vi "UTILITY Get Excel Data From Worksheet.vi"(8 "error in (no error)":errorcluster, 10 "Number of Columns":i32, 11 "template (empty)":path) -> (0 "error out":errorcluster, 3 "Array":string[][](array[string]))   [LabVIEW 2016]
uses:
  <vilib>/addons/_office/excel.llb/Excel Get Data (str).vi
  <vilib>/Utility/NIReport.llb/NI_report.lvclass
  <vilib>/Utility/NIReport.llb/Excel/NI_Excel.lvclass
  <vilib>/addons/_office/NI_ReportGenerationToolkit.lvlib
panel:
  in  "start (0, 0) 2":cluster{"start row":i32, "start column":i32}
  out "MS Office parameters out 2":T1
  # "Input the file to read"
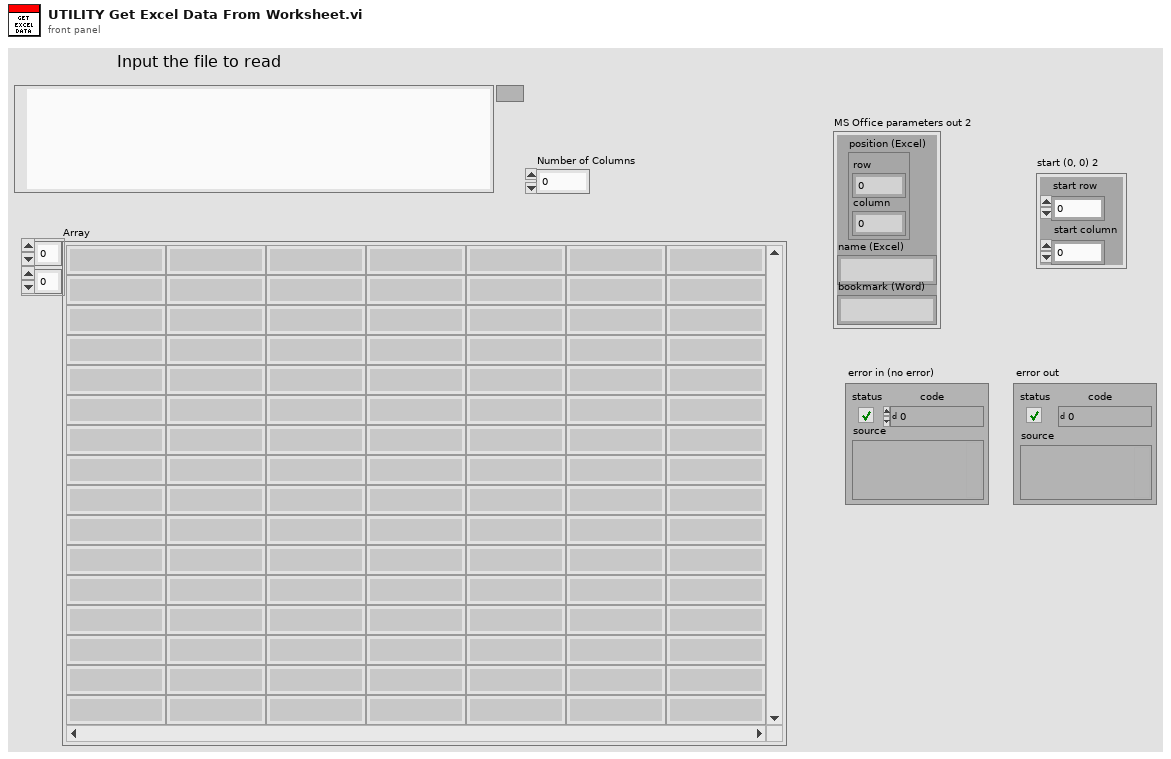
[diagram p1: front panel]
types:
  T1 = cluster{"position (Excel)":cluster{"row":i32, "column":i32}, "name (Excel)":string, "bookmark (Word)":string}
  T2 = enum16{"maximized", "minimized", "normal", "no change"}
  T3 = enum16{"Standard Report", "HTML", "Word", "Excel"}
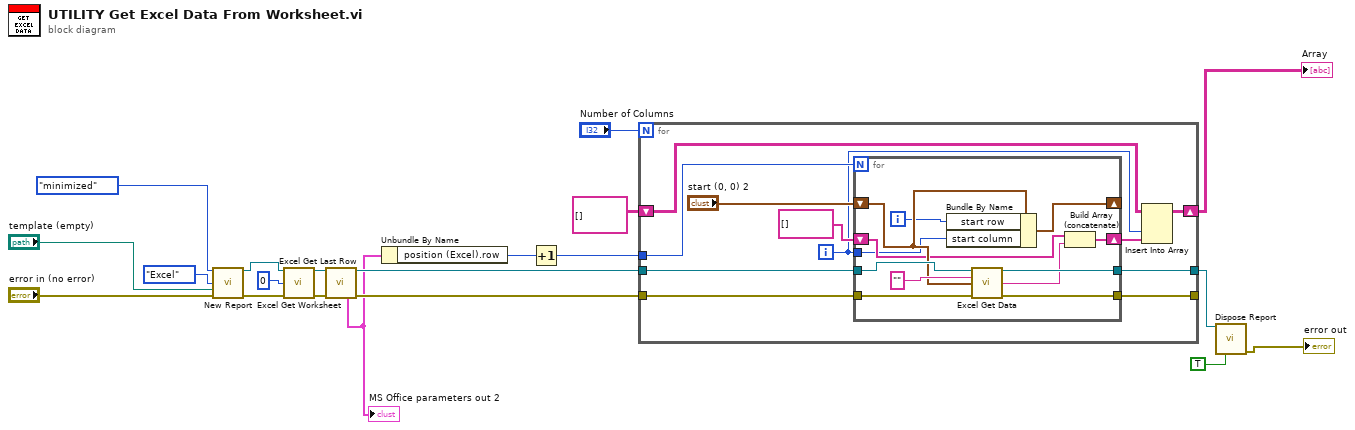
[diagram p0: block diagram]
diagram:
  n1 = call <vilib>:"New Report.vi"("window state (normal)"=T2."minimized", "report type"=T3."Excel", "template (empty)"="template (empty)", "error in (no error)"="error in (no error)") -> ("report out"=w5:refnum<class "NI_report.lvclass">, "error out"=w7:errorcluster)  [unwired: 10 in]
  n2 = call <vilib>:"Excel Get Worksheet.vi"("report in"=w5, "worksheet index (0)"=0, "error in (no error)"=w7) -> ("report out"=w8:refnum<class "NI_report.lvclass">, "error out"=w9:errorcluster)  [unwired: 11 in]
  n3 = call <vilib>:"Excel Get Last Row.vi"("report in"=w8, "error in (no error)"=w9) -> ("report out"=w11:refnum<class "NI_report.lvclass">, "MS Office parameters out"=w10:T1, "error out"=w12:errorcluster)  [unwired: 11 in]
  "MS Office parameters out 2" <- w10
  n4 = Unbundle By Name(w10) -> ("position (Excel).row"=w18:i32)
  n5 = Increment(x=w18) -> (x+1=w19:i32)
  n6 = for {
    N: "Number of Columns" -> [_]
    tunnel: w11 -> [w31]
    tunnel: w19 -> [w30]
    tunnel: w12 -> [w28]
    tunnel: [w23] -> w14
    tunnel: [w22] -> _
    shift-right: [w21] -> w15
    shift-left: string[][] [] -> [w26]
    i -> [w24]
    n7 = for {
      N: w30 -> [_]
      tunnel: w31 -> [w42]
      tunnel: [w41] -> w23
      shift-right: [w36] -> w25
      shift-left: string[] [] -> [w37]
      shift-right: [w40] -> _
      shift-left: "start (0, 0) 2" -> [w39]
      tunnel: w28 -> [w35]
      tunnel: [w34] -> w22
      tunnel: w24 -> [w33]
      i -> [w32]
      n8 = Bundle By Name(cluster=w39, "start row"=w32, "start column"=w33) -> (w40:cluster{"start row":i32, "start column":i32})
      n9 = call-poly <vilib>:"Excel Get Data.vi"("report in"=w42, "data type"="", "start (0, 0)"=w39, "error in (no error)"=w35) -> ("report out"=w41:refnum<class "NI_report.lvclass">, "data"=w38:string, "error out"=w34:errorcluster)  [unwired: 9 in]
      n10 = Build Array (concatenate)(w37, w38) -> (w36:string[])
    }
    n11 = Insert Into Array(array=w26, index (col)=w24, new element=w25) -> (w21:string[][])  [unwired: 1 in]
  }
  "Array" <- w15
  n12 = call-dynamic "Dispose Report.vi"("report in"=w14, "close report? (T)"=TRUE) -> ("error out"=→"error out":errorcluster)  [unwired: 13 in]
